vi "Magnet_GUI.vi"(10 "stop 2":refnum<vi>, 11 "GUI_cluster":T1={"Sub Panel"=refnum, "GUIdevice"="Bella_LP_Mode", "CtlRef"=refnum, "User Event in"=refnum}) -> ()   [LabVIEW 2013]
uses:
  Shared/GUI_Template/GUI_master/tcp_new_data_event.ctl
  Shared/GUI_Template/GUI_master/tcp new data cluster.ctl
  Controls/GUI_cluster.ctl
  Controls/eventtypdef1.ctl
panel:
  out "field::1":dbl caption="field (mT)" min=0.0 max=0.0
  in  "on/off":bool
  in  "curent set":u16
  out "Voltage":dbl(slide) scale=0.0..40.0
  out "CURRENT":dbl(slide) scale=0.0..250.0
  in  "stop":bool
  out "tcp data event":T2
  out "GUIdevice 1":string="StagingHexapodPI"
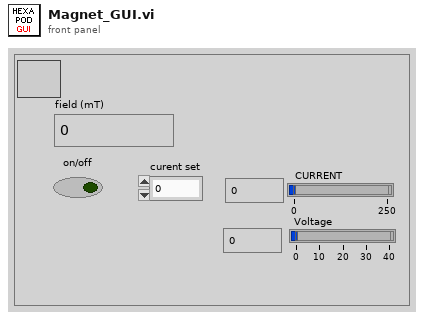
[diagram p1: front panel]
types:
  T1 = typedef "GUI_cluster.ctl" = cluster{"Sub Panel":refnum<vi>, "GUIdevice":string, "CtlRef":refnum<vi>, "User Event in":refnum<user-event>}
  T2 = typedef "tcp_new_data_event.ctl" = refnum<user-event>
  T3 = typedef "eventtypdef1.ctl" = cluster{"label":string, "Sub Panel":refnum<vi>, "CtlRef":refnum<vi>, "This VI":refnum<vi>}
  T4 = typedef "tcp new data cluster.ctl" = cluster{"EventEnum":enum16{"new data", "connection status update"}, "Device name":string}
  T5 = typedef "MagnetCluster.ctl" = cluster{"Main interlock":bool, "Flow Switch 1":bool, "Flow Switch 2":bool, "Power Supply ok":bool, "on":bool, "staging":bool, "undulator":bool, "VOLTAGE":dbl, "CURRENT":dbl, "curent set":u16}
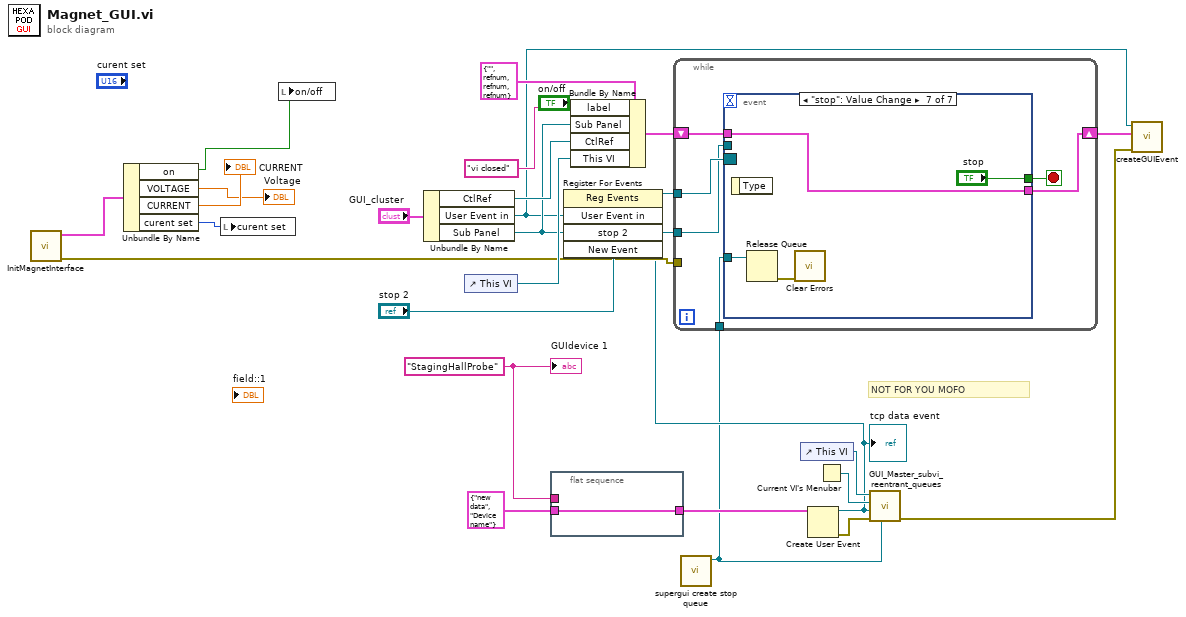
[diagram p0: block diagram]
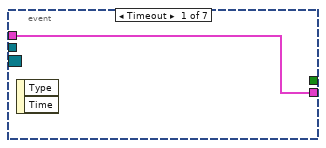
[diagram p2: hidden frame]
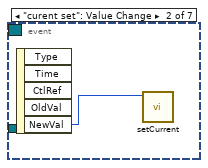
[diagram p3: hidden frame]
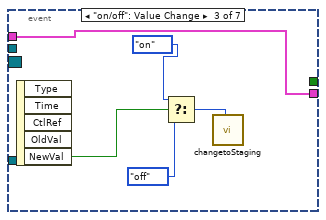
[diagram p4: hidden frame]
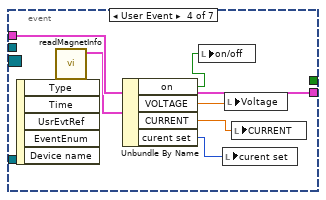
[diagram p5: hidden frame]
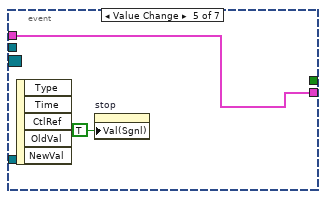
[diagram p6: hidden frame]
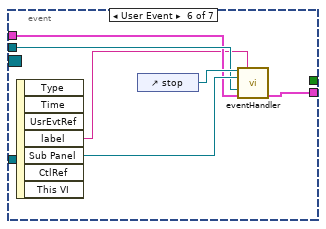
[diagram p7: hidden frame]
diagram:
  w17 = "StagingHallProbe" ("GUIdevice")
  # "NOT FOR YOU MOFO"
  n1 = call "InitMagnetInterface.vi"() -> ("error out"=w3:errorcluster, "output cluster 2"=w8:T5)  [unwired: 10 in]
  n2 = Unbundle By Name(w8) -> ("on"=w6:bool, "VOLTAGE"=→"Voltage":dbl, "CURRENT"=→"CURRENT":dbl, "curent set"=w7:u16)
  n3 = local write "curent set"(w7) -> ()
  n4 = local write "on/off"(w6) -> ()
  n5 = Unbundle By Name("GUI_cluster") -> ("CtlRef"=w19:refnum<vi>, "User Event in"=w12:refnum<user-event>, "Sub Panel"=w14:refnum<vi>)
  n6 = control-ref of="This VI"() -> (w18:refnum<vi>)
  n7 = flat-sequence {
    tunnel: T4 {"EventEnum"=enum."new data", "Device name"="Device name"} ("New Event") -> [w27]
    tunnel: [w27] -> w20
    tunnel: w17 -> [_]
    frame #0 {
    }
  }
  n8 = Bundle By Name(cluster=T3 {"label"="", "Sub Panel"=refnum, "CtlRef"=refnum, "This VI"=refnum} ("event data"), "label"="vi closed", "Sub Panel"=w14, "CtlRef"=w19, "This VI"=w18) -> (w13:T3)
  n9 = call "supergui create stop queue.vi"() -> ("STOP Queue out"=w1:refnum<queue>)  [unwired: 11 in]
  n10 = control-ref of="This VI"() -> (w26:refnum<vi>)
  n11 = Create User Event(user event datatype=w20) -> (user event=w2:refnum<user-event>, error out=w24:errorcluster)  [unwired: 1 in]
  "tcp data event" <- w2
  n12 = register-events(w12, "stop 2", w2) -> (reference out=w16:refnum<event-registration>)  [unwired: 2 in, 1 out]
  n13 = while {
    tunnel: w16 -> [w33]
    tunnel: w14 -> [w31]
    shift-right: [w29] -> w10
    shift-left: w13 -> [w30]
    tunnel: w3 -> [_]
    tunnel: w1 -> [w28]
    stop <- w32 stop-if-true
    n14 = event shown="[6] \"stop\": Value Change" {
      selector: w33 -> [_ _ _ _ _ _ _]
      dyn-events: _ -> [_ _ _ _ _ _ _]
      timeout: _ -> [_ _ _ _ _ _ _]
      tunnel: [_ _ _ _ _ _ "stop"] -> w32
      tunnel: w31 -> [_ _ _ _ _ w52 _]
      tunnel: w30 -> [w34 _ w36 w46 w48 w51 w57]
      tunnel: [w34 _ w36 w46 w48 w50 w57] -> w29
      tunnel: w28 -> [_ _ _ _ _ _ w56]
      event Timeout {
        n15 = event-data() -> ()  [unwired: 1 in, 2 out]
      }
      event "curent set": Value Change {
        n16 = event-data() -> ("NewVal"=w35:u16)  [unwired: 1 in, 4 out]
        n17 = call "setCurrent.vi"("curent set"=w35) -> ()  [unwired: 10 in, 1 out]
      }
      event "on/off": Value Change {
        n18 = event-data() -> ("NewVal"=w37:bool)  [unwired: 1 in, 4 out]
        n19 = Select(t=enum16{"off", "on", "undulator", "staging"}."on" ("cmd"), s=w37, f=enum16{"off", "on", "undulator", "staging"}."off" ("cmd")) -> (s? t:f=w40:enum16{"off", "on", "undulator", "staging"})
        n20 = call "changetoStaging.vi"("cmd"=w40) -> ()  [unwired: 10 in, 1 out]
      }
      event User Event {
        n21 = event-data() -> ()  [unwired: 1 in, 5 out]
        n22 = call "readMagnetInfo.vi"() -> ("output cluster"=w45:T5)  [unwired: 10 in, 1 out]
        n23 = Unbundle By Name(w45) -> ("on"=w44:bool, "VOLTAGE"=w43:dbl, "CURRENT"=w42:dbl, "curent set"=w41:u16)
        n24 = local write "on/off"(w44) -> ()
        n25 = local write "curent set"(w41) -> ()
        n26 = local write "Voltage"(w43) -> ()
        n27 = local write "CURRENT"(w42) -> ()
      }
      event Value Change {
        n28 = event-data() -> ()  [unwired: 1 in, 5 out]
        n29 = property on="stop" class="Bool (strict)"("Val(Sgnl)"=TRUE ("Value (Signaling)")) -> ()  [unwired: 2 in, 2 out]
      }
      event User Event {
        n30 = event-data() -> ("label"=w49:string, "Sub Panel"=w53:refnum<vi>)  [unwired: 1 in, 5 out]
        n31 = control-ref of="stop"() -> (w54:refnum<vi>)
        n32 = call "eventHandler.vi"("Boolean in"=w54, "label"=w49, "Sub Panel 2"=w53, "Sub Panel"=w52, "event data in"=w51) -> ("event data out"=w50:T3)  [unwired: 10 in]
      }
      event "stop": Value Change {
        n33 = event-data() -> ()  [unwired: 1 in, 1 out]
        n34 = Release Queue(queue=w56) -> (error out=w55:errorcluster)  [unwired: 2 in, 2 out]
        n35 = call <vilib>:"Clear Errors.vi"("error in (no error)"=w55) -> ()  [unwired: 6 in, 1 out]
      }
    }
  }
  n36 = Current VI's Menubar() -> (w25:refnum<k9>)
  n37 = call "GUI_Master_subvi_reentrant_queues.vi"("STOP Queue in"=w1, "error in (no error)"=w24, "tcp data event"=w2, "Caller menu reference"=w25, "Caller VI ref"=w26) -> ("error out"=w11:errorcluster)  [unwired: 6 in]
  n38 = call "createGUIEvent.vi"("error in (no error)"=w11, "event data"=w10, "User Event in"=w12) -> ()  [unwired: 8 in, 1 out]
  "GUIdevice 1" <- w17
